vi "Set Triggered Log State.vi"(8 "error in (no error)":errorcluster, 10 "Triggered Log State":T1, 11 "Triggered Log in":refnum<class "Triggered Log.lvclass">) -> (0 "error out":errorcluster, 3 "Triggered Log out":refnum<class "Triggered Log.lvclass">)   [LabVIEW 2012, in "Triggered Log.lvclass"]
doc: "Updates the state of the triggered log and notifies any listeners if the state has changed."
uses:
  Triggered Log.lvclass
  Triggered Log State.ctl
  Triggered Log.lvclass/Triggered Log.ctl
  Engine/Classes/Triggers/Trigger/Trigger.lvclass
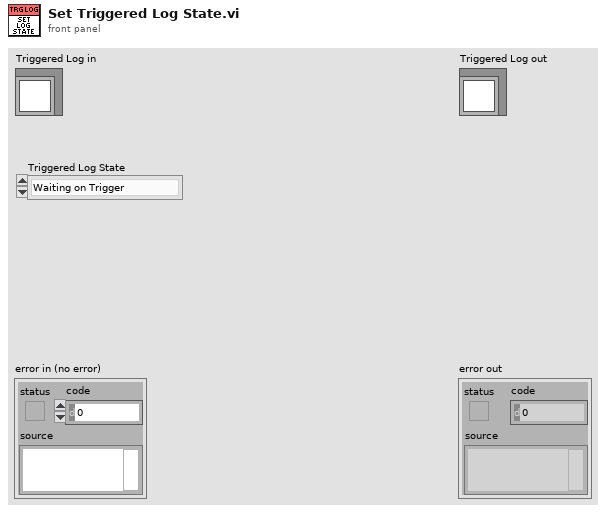
[diagram p1: front panel]
types:
  T1 = typedef "Triggered Log.lvclass/Triggered Log State.ctl" = enum16{"Waiting on Trigger", "Triggered", "Posttrigger", "Complete", "Idle", "Error"}
  T2 = typedef "Triggered Log.lvclass/Triggered Log State Change Event Registration.ctl" = cluster{"Callback":refnum<vi>, "User Data":variant}
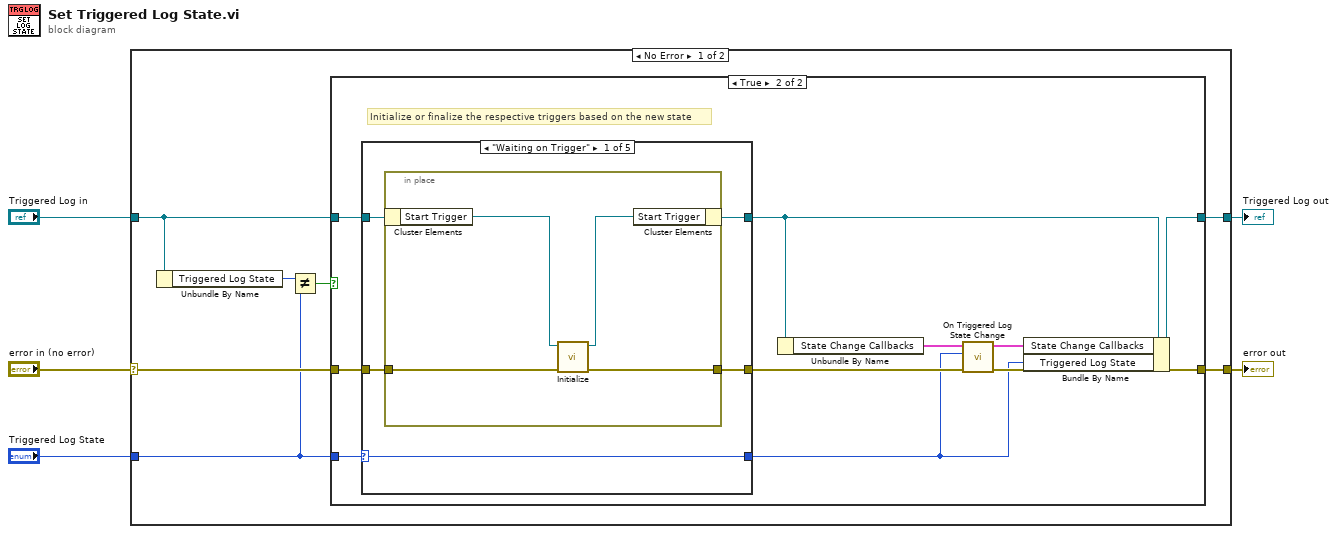
[diagram p0: block diagram]
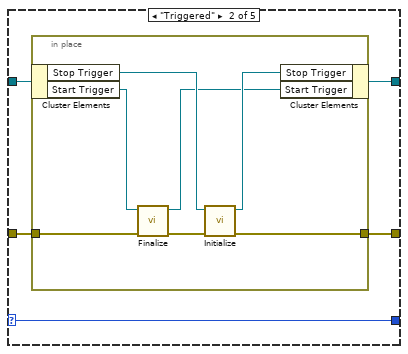
[diagram p3: hidden frame]
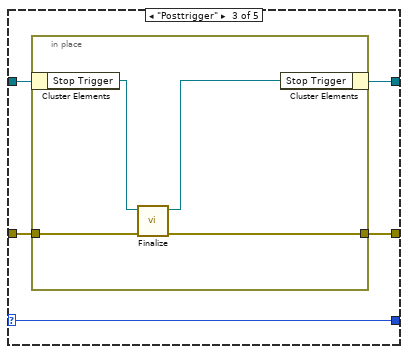
[diagram p4: hidden frame]
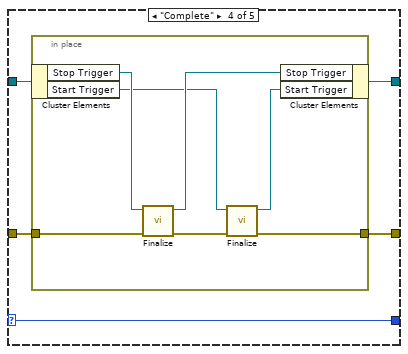
[diagram p5: hidden frame]
diagram:
  n1 = case shown="No Error" "error in (no error)" {
    selector: "error in (no error)" -> [w7 w71]
    tunnel: [w8 w71] -> w4
    tunnel: [w10 w70] -> w2
    tunnel: "Triggered Log in" -> [w9 w70]
    tunnel: "Triggered Log State" -> [w6 _]
    frame No Error {
      n2 = Unbundle By Name(w9) -> ("Triggered Log State"=w12:T1)
      n3 = Not Equal?(x=w12, y=w6) -> (x != y?=w11:bool)
      n4 = case shown="True" w11 {
        tunnel: [w14 w24] -> w10
        tunnel: w9 -> [w14 w19]
        tunnel: [w13 w23] -> w8
        tunnel: w7 -> [w13 w16]
        tunnel: w6 -> [_ w20]
        frame False {
        }
        frame True {
          # "Initialize or finalize the respective triggers based on the new state"
          n5 = case shown="\"Waiting on Trigger\"" w20 {
            selector: w20 -> [w25 w34 w46 w55 w67]
            tunnel: w19 -> [w29 w38 w50 w59 w69]
            tunnel: [w27 w36 w48 w57 w69] -> w18
            tunnel: [w26 w35 w47 w56 w68] -> w17
            tunnel: w16 -> [w28 w37 w49 w58 w68]
            tunnel: [w25 w34 w46 w55 w67] -> w15
            frame "Waiting on Trigger" {
              n6 = in-place {
                in-place-border: w28 -> [w30]
                in-place-border: [w31] -> w26
                n7 = in-place-cluster #1(w29) -> ("Start Trigger"=w33:refnum<class "Trigger.lvclass">)
                n8 = call "Initialize.vi"("error in (no error)"=w30, "Trigger in"=w33) -> ("error out"=w31:errorcluster, "Trigger out"=w32:refnum<class "Trigger.lvclass">)  [unwired: 8 in]
                n9 = in-place-cluster #1("Start Trigger"=w32) -> (w27:refnum<class "Triggered Log.lvclass">)
              }
            }
            frame "Triggered" {
              n10 = in-place {
                in-place-border: w37 -> [w42]
                in-place-border: [w43] -> w35
                n11 = in-place-cluster #2(w38) -> ("Stop Trigger"=w45:refnum<class "Trigger.lvclass">, "Start Trigger"=w40:refnum<class "Trigger.lvclass">)
                n12 = call "Finalize.vi"("error in (no error)"=w42, "Trigger in"=w40) -> ("error out"=w41:errorcluster, "Trigger out"=w39:refnum<class "Trigger.lvclass">)  [unwired: 8 in]
                n13 = call "Initialize.vi"("error in (no error)"=w41, "Trigger in"=w45) -> ("error out"=w43:errorcluster, "Trigger out"=w44:refnum<class "Trigger.lvclass">)  [unwired: 8 in]
                n14 = in-place-cluster #2("Stop Trigger"=w44, "Start Trigger"=w39) -> (w36:refnum<class "Triggered Log.lvclass">)
              }
            }
            frame "Posttrigger" {
              n15 = in-place {
                in-place-border: w49 -> [w54]
                in-place-border: [w51] -> w47
                n16 = in-place-cluster #3(w50) -> ("Stop Trigger"=w53:refnum<class "Trigger.lvclass">)
                n17 = call "Finalize.vi"("error in (no error)"=w54, "Trigger in"=w53) -> ("error out"=w51:errorcluster, "Trigger out"=w52:refnum<class "Trigger.lvclass">)  [unwired: 8 in]
                n18 = in-place-cluster #3("Stop Trigger"=w52) -> (w48:refnum<class "Triggered Log.lvclass">)
              }
            }
            frame "Complete" {
              n19 = in-place {
                in-place-border: w58 -> [w66]
                in-place-border: [w60] -> w56
                n20 = in-place-cluster #4(w59) -> ("Stop Trigger"=w65:refnum<class "Trigger.lvclass">, "Start Trigger"=w63:refnum<class "Trigger.lvclass">)
                n21 = call "Finalize.vi"("error in (no error)"=w66, "Trigger in"=w65) -> ("error out"=w61:errorcluster, "Trigger out"=w64:refnum<class "Trigger.lvclass">)  [unwired: 8 in]
                n22 = call "Finalize.vi"("error in (no error)"=w61, "Trigger in"=w63) -> ("error out"=w60:errorcluster, "Trigger out"=w62:refnum<class "Trigger.lvclass">)  [unwired: 8 in]
                n23 = in-place-cluster #4("Stop Trigger"=w64, "Start Trigger"=w62) -> (w57:refnum<class "Triggered Log.lvclass">)
              }
            }
            frame "Idle", "Error" {
            }
          }
          n24 = Unbundle By Name(w18) -> ("State Change Callbacks"=w22:T2[])
          n25 = call "On Triggered Log State Change.vi"("error in (no error)"=w17, "Log State"=w15, "Trigger Event Registrations in"=w22) -> ("error out"=w23:errorcluster, "Trigger Event Registrations out"=w21:T2[])  [unwired: 7 in]
          n26 = Bundle By Name(cluster=w18, "State Change Callbacks"=w21, "Triggered Log State"=w15) -> (w24:refnum<class "Triggered Log.lvclass">)
        }
      }
    }
    frame Error {
    }
  }
  "error out" <- w4
  "Triggered Log out" <- w2
